vi "Configure Track.vi"(8 "error in (no error)":errorcluster, 9 "Track Mode (0: ON)":i32(ring) items=["ON", "OFF", "Inverted"], 10 "Source Channel (1: 1)":i32(ring)=1 items=["1"=1, "2"=2], 11 "VISA resource name":refnum<visa-resource-name>) -> (0 "error out":errorcluster, 3 "VISA resource name out":refnum<visa-resource-name>)   [LabVIEW 2015, in "Agilent 3352X Series.lvlib"]
doc: "Causes channels 1 and 2 of a two channel waveform generator to output the same signal, or an inverted polarity signal.\n\n<b>Note</b>:\nOnly valid on the 2-channel instrument."
uses:
  <instrlib>/Agilent 3352X Series/Agilent 3352X Series.lvlib
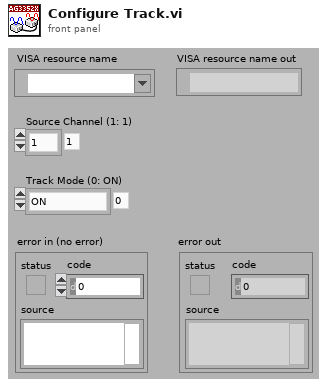
[diagram p1: front panel]
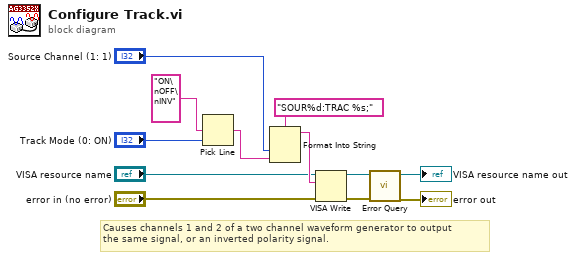
[diagram p0: block diagram]
diagram:
  # "Causes channels 1 and 2 of a two channel waveform generator to output \nthe same signal, or an inverted polarity signal."
  n1 = Pick Line(multi-line string="ON\nOFF\nINV", line index="Track Mode (0: ON)") -> (output string=w8:string)  [unwired: 1 out]
  n2 = Format Into String(format string="SOUR%d:TRAC %s;", "Source Channel (1: 1)", w8) -> (resulting string=w7:string)  [unwired: 2 in, 1 out]
  n3 = VISA Write(VISA resource name="VISA resource name", write buffer=w7, error in (no error)="error in (no error)") -> (VISA resource name out=w4:refnum<visa-resource-name>, error out=w3:errorcluster)  [unwired: 1 out]
  n4 = call <instrlib>:"Error Query.vi"("error in (no error)"=w3, "VISA resource name"=w4) -> ("error out"=→"error out":errorcluster, "VISA resource name out"=→"VISA resource name out":refnum<visa-resource-name>)  [unwired: 8 out]
